vi "Exp04_ComplementaryFilter.vi"() -> ()   [LabVIEW 2019]
uses:
  <vilib>/myRIO/Instrument Drivers/Onboard IO/I2C/typedefs/I2C User Configuration.ctl
  <vilib>/myRIO/Instrument Drivers/Onboard IO/I2C/typedefs/I2C Transfer Rate.ctl
  <vilib>/Platform/TimedLoop/XDataNode/timing_clust.ctl
  <vilib>/Platform/TimedLoop/XDataNode/nitl_modes.ctl
  <vilib>/Platform/TimedLoop/XDataNode/wakeup.ctl
  <vilib>/Utility/error.llb/Error Cluster From Error Code.vi
  <vilib>/myRIO/Common/Instrument Driver Framework/myRIO v1.0/I2C/vis/myRIO v1.0 Configure I2C.vi
  <vilib>/myRIO/Common/Instrument Driver Framework/myRIO v1.0/I2C/vis/myRIO v1.0 Write I2C.vi
  <vilib>/myRIO/Common/Instrument Driver Framework/myRIO v1.0/I2C/vis/myRIO v1.0 Read I2C.vi
  <vilib>/Platform/TimedLoop/XDataNode/XDataNode.xnode
  <vilib>/myRIO/Instrument Drivers/Onboard IO/I2C/I2C.lvlib
  <vilib>/Platform/TimedLoop/XDataNode/XDNodeRunTimeDep.lvlib
panel:
  out "Angle":dbl[][](graph)
  out "gyro angle":dbl
  in  "zero":bool
  in  "initial bias":i16
  out "angular velocity":dbl
  out "acc angle":dbl
  out "Gyro Z":i16
  out "Gyro X":i16
  out "Gyro Y":i16
  out "Acc Z":i16
  out "Temperature":dbl
  out "Acc Y":i16
  out "Acc X":i16
  in  "stop":bool
  out "error out":errorcluster
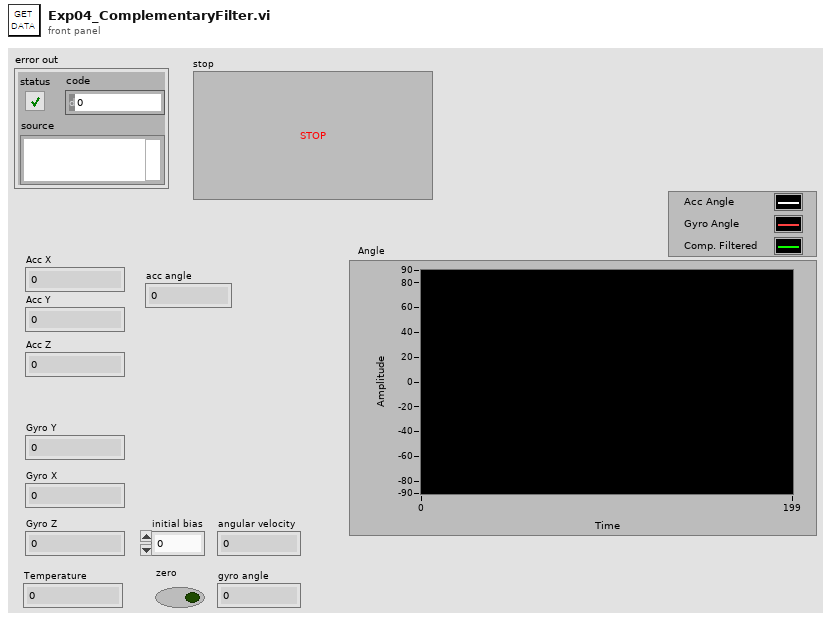
[diagram p1: front panel]
types:
  T1 = typedef "I2C.lvlib/I2C User Configuration.ctl" = cluster{"I2C Transfer Rate":T2}
  T2 = typedef "I2C.lvlib/I2C Transfer Rate.ctl" = enum16{"Standard mode (100 kbps)", "Fast mode (400 kbps)"}
  T3 = typedef "I2C.lvlib/I2C Reference.ctl" = cluster{"myRIO Reference":T4, "I2C Channels Enum":T8, "I2C Configuration":T9}
  T4 = typedef "myRIO Generic Hardware Reference.ctl" = cluster{"myRIO Model":T5, "myRIO Hardware Reference":T6}
  T5 = typedef "Hardware Version Enum.ctl" = enum16{"Unknown", "myRIO-1900", "myRIO-1950", "roboRIO", "NI ELVIS RIO CM", "ELVIS III"}
  T6 = typedef "myRIO v1.0 Reference.ctl" = cluster{"Generic FPGA Reference":T7, "Allow multiple opens":bool}
  T7 = typedef "Generic FPGA Reference.ctl" = refnum<k20>
  T8 = typedef "I2C Channels Enum.ctl" = enum16{"Not Connected", "A/I2C", "B/I2C", "I2C/I2C"}
  T9 = typedef "I2C.lvlib/I2C Configuration.ctl" = cluster{"I2C Transfer Rate":T2}
  T10 = typedef "XDNodeRunTimeDep.lvlib/timing_clust.ctl" = cluster{"Expected End [f-1]":u64, "Actual End [f-1]":u64, "Finished Late? [f-1]":bool, "Expected End [i-1]":u64, "Actual End [i-1]":u64, "Finished Late? [i-1]":bool, "Expected Start [i]":u64, "Actual Start [i]":u64, "Expected Start [f]":u64, "Actual Start [f]":u64, "Source Name":string, "Structure Name":string, "Period":i64, "Deadline":i64, "Offset":i64, "Start":i64, "Priority":i32, "Timeout":i32, "Mode":T11, "Wakeup Reason":T12, "Error":errorcluster, "Source Type":string, "Secondary Source Type":string, "Global End Time":u64, "Global Start Time":u64, "Frame Duration":u64, "Iteration Duration":u64, "Assigned CPU":i32, "I/O Scan Engine Mode":u32}
  T11 = typedef "XDNodeRunTimeDep.lvlib/nitl_modes.ctl" = enum32{"No Change", "Process missed periods, maintain original phase", "Discard missed periods, maintain original phase", "Process missed periods, ignore original phase", "Discard missed periods, ignore original phase"}
  T12 = typedef "XDNodeRunTimeDep.lvlib/wakeup.ctl" = enum32{"Normal", "Aborted", "Asynchronous wakeup", "Timing source error", "Timed loop error", "Timeout"}
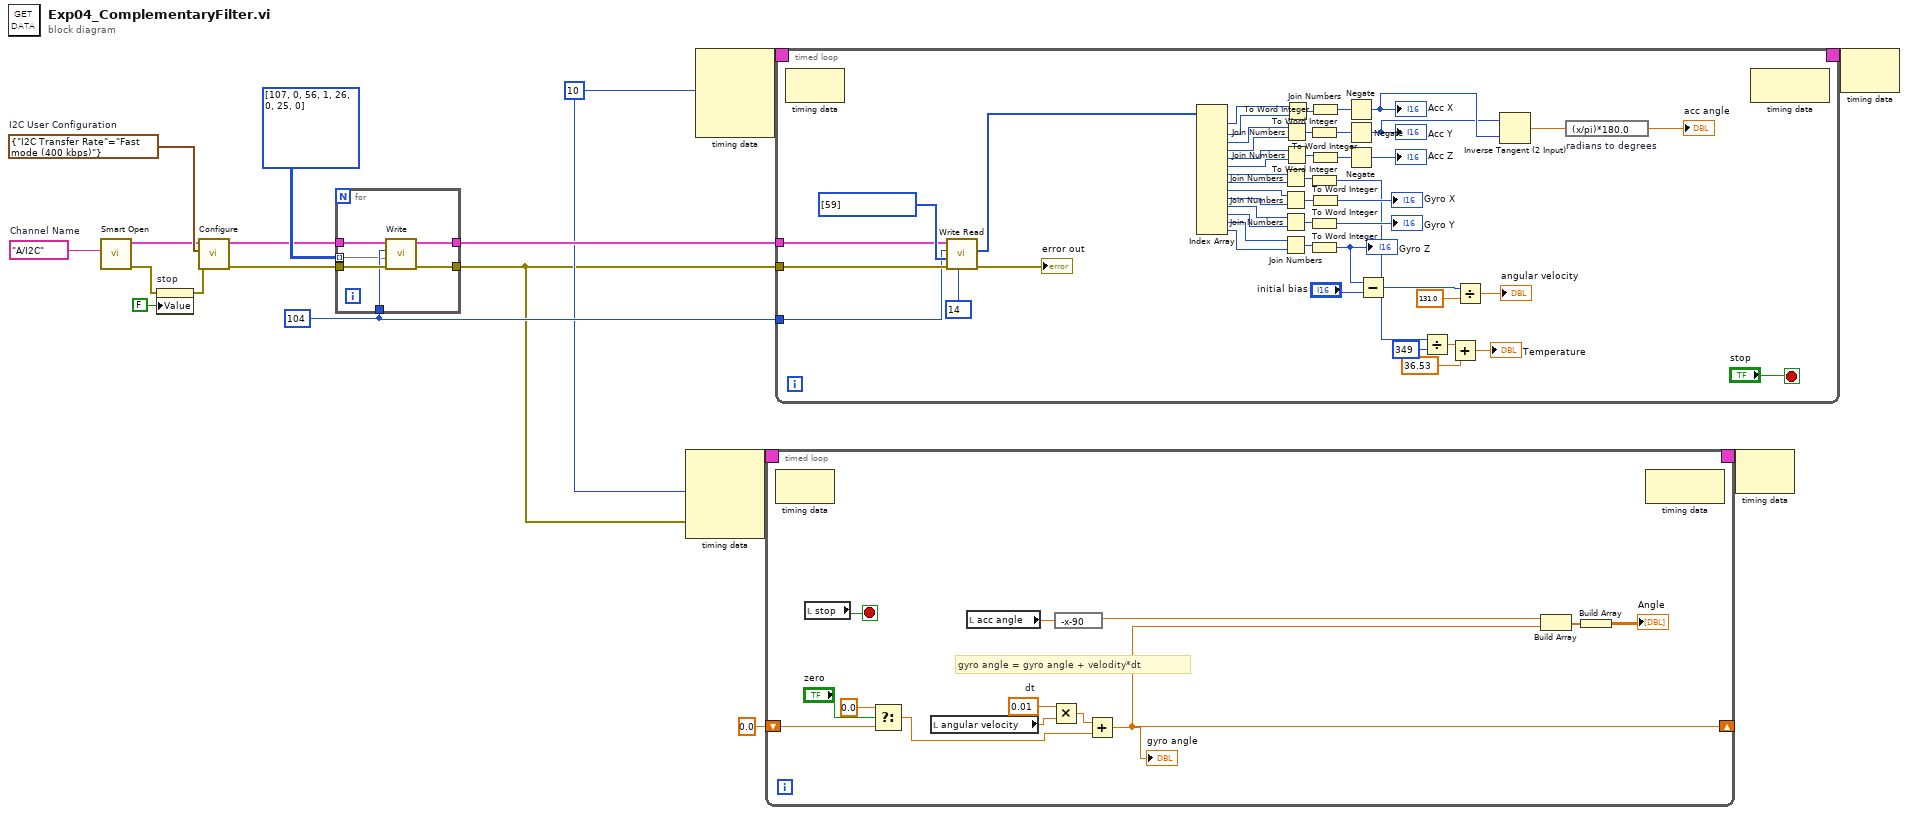
[diagram p0: block diagram]
diagram:
  w14 = u8 104 ("Slave Address (7-bit)")
  w2 = i64 10 ("Period")
  w17 = T1 {"I2C Transfer Rate"=enum."Fast mode (400 kbps)"}  # I2C User Configuration
  w18 = tag "A/I2C"  # Channel Name
  n1 = call <vilib>:"Smart Open.vi"("Channel Name"=w18) -> ("error out"=w5:errorcluster, "I2C Ref Out"=w16:T3)  [unwired: 9 in]
  n2 = property on="stop" class="Bool (strict)"(error in=w5, "Value"=FALSE ("stop")) -> (error out=w3:errorcluster)  [unwired: 1 in, 1 out]
  n3 = call <vilib>:"Configure.vi"("error in (no error)"=w3, "I2C User Configuration"=w17, "I2C Ref In"=w16) -> ("error out"=w9:errorcluster, "I2C Ref Out"=w10:T3)  [unwired: 7 in]
  n4 = for {
    tunnel: w14 -> [w20]
    tunnel: w10 -> [w24]
    tunnel: [w21] -> w15
    tunnel: w9 -> [w23]
    tunnel: [w22] -> w1
    tunnel: u8[][] [[107, 0], [56, 1], [26, 0], [25, 0]] ("Bytes to Write") -> [w19] mode=indexing
    n5 = call <vilib>:"Write.vi"("error in (no error)"=w23, "Bytes to Write"=w19, "Slave Address (7-bit)"=w20, "I2C Ref In"=w24) -> ("error out"=w22:errorcluster, "I2C Ref Out"=w21:T3)  [unwired: 6 in]
  }
  n6 = node-c288(w2, w1) -> (w8:T10)  [unwired: 2 in]
  n7 = node-c288(w2) -> (w13:T10)  [unwired: 3 in]
  n8 = timed-loop {
    timing: w8 -> [_]
    timing-out: [_] -> w7
    shift-right: [w25] -> _
    shift-left: 0.0 -> [w32]
    stop <- w30 stop-if-true
    w36 = 0.01  # dt
    # "gyro angle = gyro angle + velodity*dt"
    n9 = node-c288() -> ()  [unwired: 1 in, 1 out]
    n10 = local read "stop"() -> (w30:bool)
    n11 = Select(t=0.0, s="zero", f=w32) -> (s? t:f=w31:dbl)
    n12 = local read "angular velocity"() -> (w37:dbl)
    n13 = local read "acc angle"() -> (w27:dbl)
    n14 = Multiply(x=w36, y=w37) -> (x*y=w35:dbl)
    n15 = expression code="-x-90"(w27) -> (w26:dbl)
    n16 = Add(x=w35, y=w31) -> (x+y=w25:dbl)
    "gyro angle" <- w25
    n17 = Build Array(w26, w25) -> (w29:dbl[])
    n18 = Build Array(w29) -> (→"Angle":dbl[][])
    n19 = node-c288() -> ()  [unwired: 1 in, 1 out]
  }
  n20 = timed-loop {
    timing: w13 -> [_]
    timing-out: [_] -> w12
    tunnel: w1 -> [w85]
    tunnel: w15 -> [w84]
    tunnel: w14 -> [w83]
    stop <- "stop" stop-if-true
    n21 = node-c288() -> ()  [unwired: 1 in, 1 out]
    n22 = call <vilib>:"Write Read.vi"("Byte Count"=u32 14, "error in (no error)"=w85, "Bytes to Write"=u8[] [59], "Slave Address (7-bit)"=w83, "I2C Ref In"=w84) -> ("error out"=→"error out":errorcluster, "Bytes Read"=w53:u8[])  [unwired: 3 in, 1 out]
    n23 = Index Array(array=w53) -> (element #1=w81:u8, element #2=w80:u8, element #3=w79:u8, element #4=w78:u8, element #5=w77:u8, element #6=w76:u8, element #7=w75:u8, element #8=w74:u8, element #9=w73:u8, element #10=w72:u8, element #11=w71:u8, element #12=w70:u8, element #13=w69:u8, element #14=w68:u8)  [unwired: 14 in]
    n24 = Join Numbers(hi=w75, lo=w74) -> ((hi.lo)=w64:u16)
    n25 = Join Numbers(hi=w73, lo=w72) -> ((hi.lo)=w63:u16)
    n26 = Join Numbers(hi=w71, lo=w70) -> ((hi.lo)=w62:u16)
    n27 = Join Numbers(hi=w69, lo=w68) -> ((hi.lo)=w61:u16)
    n28 = Join Numbers(hi=w79, lo=w78) -> ((hi.lo)=w66:u16)
    n29 = Join Numbers(hi=w77, lo=w76) -> ((hi.lo)=w65:u16)
    n30 = Join Numbers(hi=w81, lo=w80) -> ((hi.lo)=w67:u16)
    n31 = To Word Integer(number=w66) -> (16bit integer=w48:i16)
    n32 = To Word Integer(number=w64) -> (16bit integer=w58:i16)
    n33 = To Word Integer(number=w62) -> (16bit integer=→"Gyro Y":i16)
    n34 = To Word Integer(number=w61) -> (16bit integer=w42:i16)
    "Gyro Z" <- w42
    n35 = To Word Integer(number=w67) -> (16bit integer=w50:i16)
    n36 = To Word Integer(number=w65) -> (16bit integer=w47:i16)
    n37 = To Word Integer(number=w63) -> (16bit integer=→"Gyro X":i16)
    n38 = Negate(x=w50) -> (-x=w49:i16)
    "Acc X" <- w49
    n39 = Negate(x=w48) -> (-x=w45:i16)
    "Acc Y" <- w45
    n40 = Negate(x=w47) -> (-x=→"Acc Z":i16)
    n41 = Subtract(x=w42, y="initial bias") -> (x-y=w40:i16)
    n42 = Divide(x=w58, y=i16 349) -> (x/y=w56:dbl)
    n43 = Add(x=w56, y=36.53) -> (x+y=→"Temperature":dbl)
    n44 = Divide(x=w40, y=131.0) -> (x/y=→"angular velocity":dbl)
    n45 = Inverse Tangent (2 Input)(1:w49, 2:w45) -> (0:w52:dbl)
    n46 = expression code="(x/pi)*180.0" "radians to degrees"(w52) -> (→"acc angle":dbl)
    n47 = node-c288() -> ()  [unwired: 1 in, 1 out]
  }
  n48 = node-c288(w7) -> ()  [unwired: 1 out]
  n49 = node-c288(w12) -> ()  [unwired: 1 out]
